vi "AE Lunch_KFCUpdate.vi"(11 "Array of AEs":T1=[{"Name"="Peng", "Go?"=TRUE, "Which batch?"=enum."Anything"}, {"Name"="Xue Sheng", "Go?"=TRUE, "Which batch?"=enum."Anything"}, {"Name"="Denny", "Go?"=TRUE, "Which batch?"=enum."Anything"}, {"Name"="Wilbur", "Go?"=TRUE, "Which batch?"=enum."Anything"}, {"Name"="Hafiz", "Go?"=TRUE, "Which batch?"=enum."Anything"}, {"Name"="James", "Go?"=TRUE, "Which batch?"=enum."Anything"}, {"Name"="Sharath", "Go?"=TRUE, "Which batch?"=enum."Anything"}, {"Name"="Habib", "Go?"=TRUE, "Which batch?"=enum."Anything"}, {"Name"="Stephen", "Go?"=TRUE, "Which batch?"=enum."Anything"}]) -> (1 "Not Going":string[](array[string]), 2 "Second Batch":string[](array[string]), 3 "First Batch":string[](array[string]), 4 "Second Batch Food":string, 5 "First Batch Food":string)   [LabVIEW 2016]
uses:
  Array AE Data.ctl
  AE Data.ctl
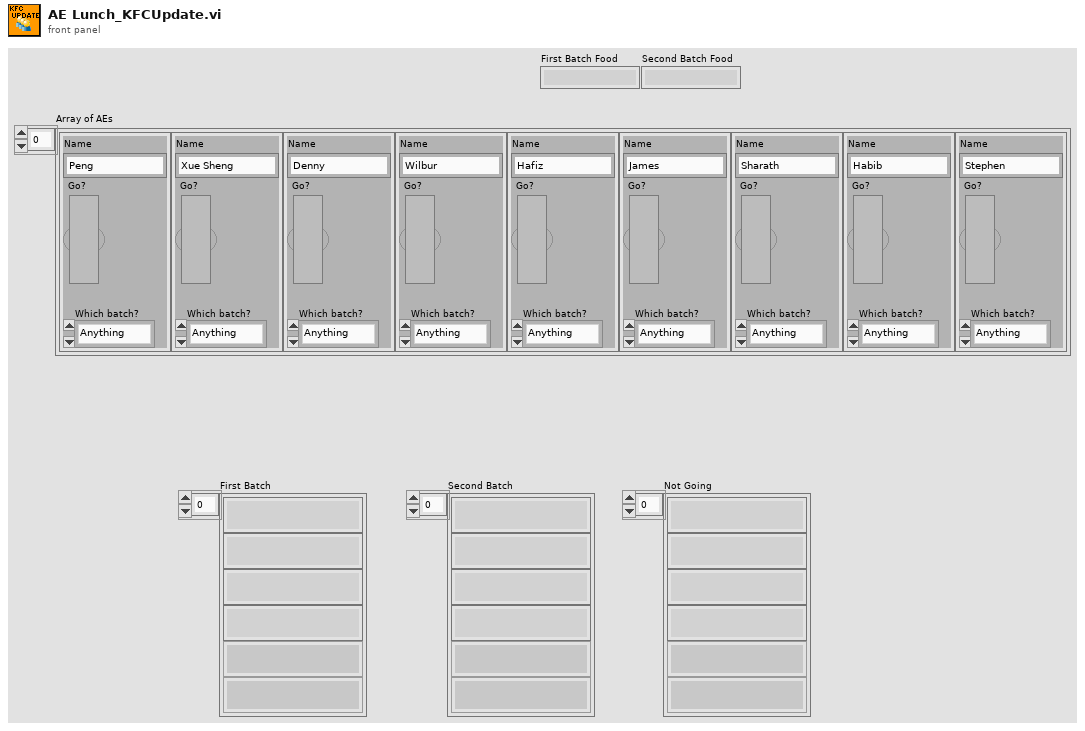
[diagram p1: front panel]
types:
  T1 = typedef "Array AE Data.ctl" = T2[]
  T2 = typedef "AE Data.ctl" = cluster{"Name":string, "Go?":bool, "Which batch?":enum16{"Anything", "First", "Second"}}
  T3 = cluster{"Name":string, "Go?":bool, "Which batch?":enum16{"Anything", "First", "Second"}, "KFC":enum16{"Anything", "KFC", "No KFC", ""}}
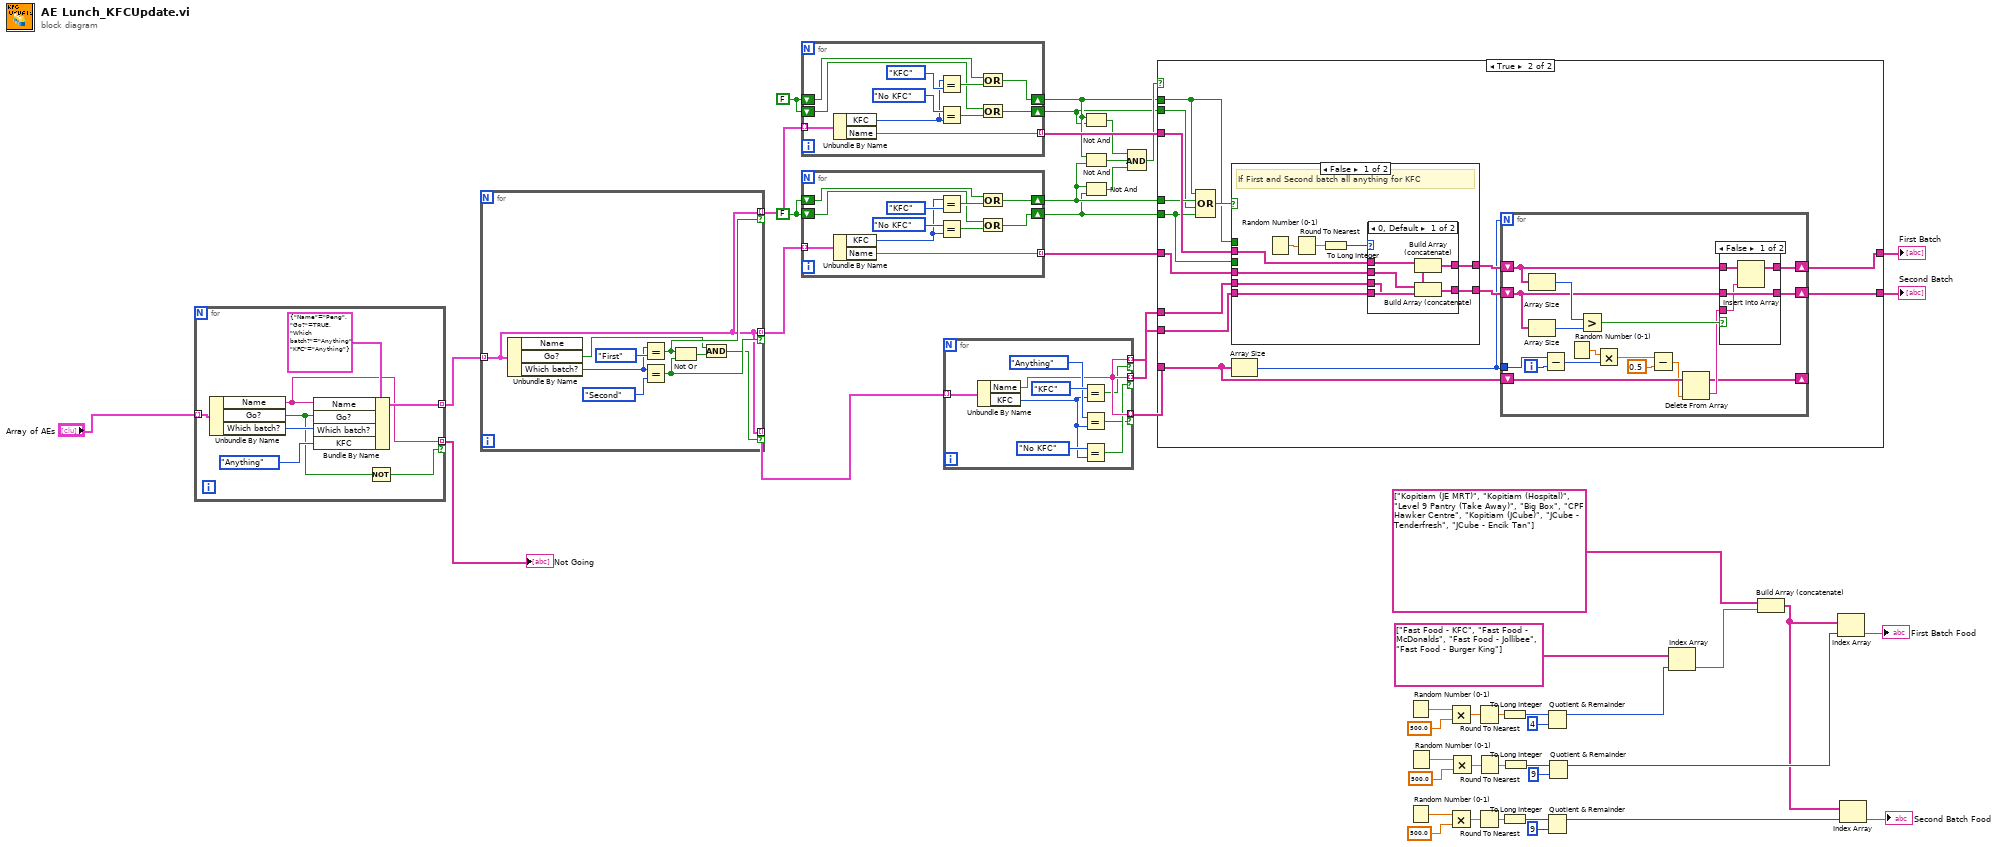
[diagram p0: block diagram]
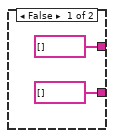
[diagram p2: hidden frame]
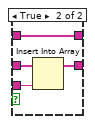
[diagram p3: hidden frame]
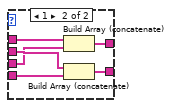
[diagram p4: hidden frame]
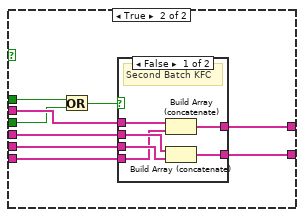
[diagram p5: hidden frame]
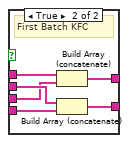
[diagram p6: hidden frame]
diagram:
  w48 = FALSE
  w49 = FALSE
  n1 = for {
    tunnel: [w54] -> w30 mode=indexing
    tunnel: "Array of AEs" -> [w58] mode=indexing
    tunnel: [w51] -> w28 mode=indexing if=w52
    n2 = Unbundle By Name(w58) -> ("Name"=w51:string, "Go?"=w53:bool, "Which batch?"=w57:enum16{"Anything", "First", "Second"})
    n3 = Bundle By Name(cluster=T3 {"Name"="Peng", "Go?"=TRUE, "Which batch?"=enum."Anything", "KFC"=enum."Anything"} ("AE"), "Name"=w51, "Go?"=w53, "Which batch?"=w57, "KFC"=enum16{"Anything", "KFC", "No KFC", ""}."Anything") -> (w54:T3)
    n4 = Not(x=w53) -> (.not. x?=w52:bool)
  }
  "Not Going" <- w28
  n5 = for {
    tunnel: w30 -> [w59] mode=indexing
    tunnel: [w59] -> w36 mode=indexing if=w60
    tunnel: [w59] -> w50 mode=indexing if=w64
    tunnel: [w59] -> w47 mode=indexing if=w63
    n6 = Unbundle By Name(w59) -> ("Go?"=w61:bool, "Which batch?"=w66:enum16{"Anything", "First", "Second"})  [unwired: 1 out]
    n7 = Equal?(x=w66, y=enum16{"Anything", "First", "Second"}."First" ("Which batch?")) -> (x = y?=w64:bool)
    n8 = Equal?(x=w66, y=enum16{"Anything", "First", "Second"}."Second" ("Which batch?")) -> (x = y?=w63:bool)
    n9 = Not Or(1:w63, 2:w64) -> (0:w62:bool)
    n10 = And(x=w61, y=w62) -> (x .and. y?=w60:bool)
  }
  n11 = for {
    tunnel: w50 -> [w77] mode=indexing
    tunnel: [w68] -> w46 mode=indexing
    shift-right: [w74] -> w40
    shift-left: w49 -> [w76]
    shift-right: [w70] -> w32
    shift-left: w49 -> [w69]
    n12 = Unbundle By Name(w77) -> ("KFC"=w72:enum16{"Anything", "KFC", "No KFC", ""}, "Name"=w68:string)
    n13 = Equal?(x=w72, y=enum16{"Anything", "KFC", "No KFC", ""}."KFC" ("KFC")) -> (x = y?=w75:bool)
    n14 = Equal?(x=enum16{"Anything", "KFC", "No KFC", ""}."No KFC" ("KFC"), y=w72) -> (x = y?=w71:bool)
    n15 = Or(x=w76, y=w75) -> (x .or. y?=w74:bool)
    n16 = Or(x=w69, y=w71) -> (x .or. y?=w70:bool)
  }
  n17 = for {
    tunnel: w47 -> [w88] mode=indexing
    tunnel: [w79] -> w45 mode=indexing
    shift-right: [w85] -> w39
    shift-left: w48 -> [w87]
    shift-right: [w81] -> w31
    shift-left: w48 -> [w80]
    n18 = Unbundle By Name(w88) -> ("KFC"=w83:enum16{"Anything", "KFC", "No KFC", ""}, "Name"=w79:string)
    n19 = Equal?(x=w83, y=enum16{"Anything", "KFC", "No KFC", ""}."KFC" ("KFC")) -> (x = y?=w86:bool)
    n20 = Equal?(x=enum16{"Anything", "KFC", "No KFC", ""}."No KFC" ("KFC"), y=w83) -> (x = y?=w82:bool)
    n21 = Or(x=w87, y=w86) -> (x .or. y?=w85:bool)
    n22 = Or(x=w80, y=w82) -> (x .or. y?=w81:bool)
  }
  n23 = for {
    tunnel: w36 -> [w98] mode=indexing
    tunnel: [w93] -> w35 mode=indexing if=w92
    tunnel: [w93] -> w34 mode=indexing if=w91
    tunnel: [w93] -> w33 mode=indexing if=w90
    n24 = Unbundle By Name(w98) -> ("Name"=w93:string, "KFC"=w94:enum16{"Anything", "KFC", "No KFC", ""})
    n25 = Equal?(x=enum16{"Anything", "KFC", "No KFC", ""}."KFC" ("KFC"), y=w94) -> (x = y?=w92:bool)
    n26 = Equal?(x=enum16{"Anything", "KFC", "No KFC", ""}."Anything" ("KFC"), y=w94) -> (x = y?=w90:bool)
    n27 = Equal?(x=enum16{"Anything", "KFC", "No KFC", ""}."No KFC" ("KFC"), y=w94) -> (x = y?=w91:bool)
  }
  n28 = Not And(1:w32, 2:w40) -> (0:w44:bool)
  n29 = Not And(1:w39, 2:w40) -> (0:w42:bool)
  n30 = Not And(1:w31, 2:w39) -> (0:w43:bool)
  n31 = Compound Arithmetic op=AND(w44, w42, w43) -> (w41:bool)
  n32 = case shown="True" w41 {
    tunnel: w46 -> [_ w115]
    tunnel: w45 -> [_ w114]
    tunnel: w35 -> [_ w113]
    tunnel: w40 -> [_ w105]
    tunnel: w39 -> [_ w107]
    tunnel: [string[] [] w111] -> w38
    tunnel: [string[] [] w108] -> w37
    tunnel: w34 -> [_ w103]
    tunnel: w33 -> [_ w104]
    tunnel: w32 -> [_ w102]
    tunnel: w31 -> [_ w101]
    frame False {
    }
    frame True {
      n33 = Compound Arithmetic op=OR(w105, w107, w102, w101) -> (w106:bool)
      n34 = case "Case" shown="False" w106 {
        tunnel: w115 -> [w148 w170]
        tunnel: w114 -> [w149 w168]
        tunnel: w113 -> [w147 w166]
        tunnel: [w146 w169] -> w112
        tunnel: [w145 w167] -> w110
        tunnel: w105 -> [_ w164]
        tunnel: w103 -> [w144 w165]
        tunnel: w101 -> [_ w163]
        frame False {
          # "If First and Second batch all anything for KFC"
          n35 = Random Number (0-1)() -> (number: 0 to 1=w143:dbl)
          n36 = Round To Nearest(number=w143) -> (nearest integer value=w142:dbl)
          n37 = To Long Integer(number=w142) -> (32bit integer=w141:i32)
          n38 = case shown="0, Default" w141 {
            tunnel: w149 -> [w154 w161]
            tunnel: w148 -> [w155 w160]
            tunnel: w147 -> [w152 w159]
            tunnel: [w151 w158] -> w146
            tunnel: [w150 w157] -> w145
            tunnel: w144 -> [w153 w156]
            frame 0, Default {
              n39 = Build Array (concatenate)(w155, w153) -> (w151:string[])
              n40 = Build Array (concatenate)(w154, w152) -> (w150:string[])
            }
            frame 1 {
              n41 = Build Array (concatenate)(w160, w159) -> (w158:string[])
              n42 = Build Array (concatenate)(w161, w156) -> (w157:string[])
            }
          }
        }
        frame True {
          n43 = Or(x=w164, y=w163) -> (x .or. y?=w162:bool)
          n44 = case shown="False" w162 {
            tunnel: w170 -> [w176 w182]
            tunnel: [w172 w180] -> w169
            tunnel: w168 -> [w175 w181]
            tunnel: [w174 w178] -> w167
            tunnel: w166 -> [w173 w179]
            tunnel: w165 -> [w171 w177]
            frame False {
              # "Second Batch KFC"
              n45 = Build Array (concatenate)(w176, w171) -> (w172:string[])
              n46 = Build Array (concatenate)(w175, w173) -> (w174:string[])
            }
            frame True {
              # "First Batch KFC"
              n47 = Build Array (concatenate)(w182, w179) -> (w180:string[])
              n48 = Build Array (concatenate)(w181, w177) -> (w178:string[])
            }
          }
        }
      }
      n49 = Array Size(array=w104) -> (size(s)=w109:i32)
      n50 = for {
        N: w109 -> [_]
        shift-right: [w123] -> w111
        shift-left: w112 -> [w127]
        shift-right: [w122] -> w108
        shift-left: w110 -> [w128]
        shift-right: [w124] -> _
        shift-left: w104 -> [w126]
        tunnel: w109 -> [w121]
        i -> [w120]
        n51 = Array Size(array=w127) -> (size(s)=w131:i32)
        n52 = Array Size(array=w128) -> (size(s)=w130:i32)
        n53 = Subtract(x=w121, y=w120) -> (x-y=w119:i32)
        n54 = Random Number (0-1)() -> (number: 0 to 1=w132:dbl)
        n55 = Greater?(x=w131, y=w130) -> (0:w129:bool)
        n56 = Multiply(x=w132, y=w119) -> (x*y=w118:dbl)
        n57 = Subtract(x=w118, y=0.5) -> (x-y=w116:dbl)
        n58 = Delete From Array(array=w126, index=w116) -> (deleted portion=w125:string, array with subset deleted=w124:string[])  [unwired: 1 in]
        n59 = case shown="False" w129 {
          tunnel: w128 -> [w135 w140]
          tunnel: w127 -> [w136 w139]
          tunnel: w125 -> [w133 w137]
          tunnel: [w134 w139] -> w123
          tunnel: [w135 w138] -> w122
          frame False {
            n60 = Insert Into Array(array=w136, new element=w133) -> (w134:string[])  [unwired: 1 in]
          }
          frame True {
            n61 = Insert Into Array(array=w140, new element=w137) -> (w138:string[])  [unwired: 1 in]
          }
        }
      }
    }
  }
  "First Batch" <- w38
  "Second Batch" <- w37
  n62 = Random Number (0-1)() -> (number: 0 to 1=w27:dbl)
  n63 = Random Number (0-1)() -> (number: 0 to 1=w10:dbl)
  n64 = Random Number (0-1)() -> (number: 0 to 1=w16:dbl)
  n65 = Multiply(x=w27, y=500.0) -> (x*y=w25:dbl)
  n66 = Multiply(x=w10, y=500.0) -> (x*y=w8:dbl)
  n67 = Multiply(x=w16, y=500.0) -> (x*y=w18:dbl)
  n68 = Round To Nearest(number=w25) -> (nearest integer value=w24:dbl)
  n69 = Round To Nearest(number=w8) -> (nearest integer value=w7:dbl)
  n70 = Round To Nearest(number=w18) -> (nearest integer value=w19:dbl)
  n71 = To Long Integer(number=w24) -> (32bit integer=w23:i32)
  n72 = To Long Integer(number=w7) -> (32bit integer=w6:i32)
  n73 = To Long Integer(number=w19) -> (32bit integer=w20:i32)
  n74 = Quotient & Remainder(x=w23, y=4) -> (x-y*floor(x/y)=w14:i32)  [unwired: 1 out]
  n75 = Quotient & Remainder(x=w6, y=9) -> (x-y*floor(x/y)=w3:i32)  [unwired: 1 out]
  n76 = Quotient & Remainder(x=w20, y=9) -> (x-y*floor(x/y)=w11:i32)  [unwired: 1 out]
  n77 = Index Array(array=string[] ["Fast Food - KFC", "Fast Food - McDonalds", "Fast Food - Jollibee", "Fast Food - Burger King"], index=w14) -> (element=w12:string)
  n78 = Build Array (concatenate)(string[] ["Kopitiam (JE MRT)", "Kopitiam (Hospital)", "Level 9 Pantry (Take Away)", "Big Box", "CPF Hawker Centre", "Kopitiam (JCube)", "JCube - Tenderfresh", "JCube - Encik Tan"], w12) -> (w4:string[])
  n79 = Index Array(array=w4, index=w11) -> (element=→"First Batch Food":string)
  n80 = Index Array(array=w4, index=w3) -> (element=→"Second Batch Food":string)
